vi "GLOBAL_odour_stimuli.vi"() -> ()   [LabVIEW 2016]
panel:
  in  "Odour stimuli":T1(array[cluster])=[{"Name"="UNNAMED2", "Bottles"=[5, 3], "Conc."=1.0, "Unit"=enum."ppm", "Duration"=250.0}, {"Name"="UNNAMED2", "Bottles"=[5, 3], "Conc."=1.0, "Unit"=enum."ppm", "Duration"=250.0}]
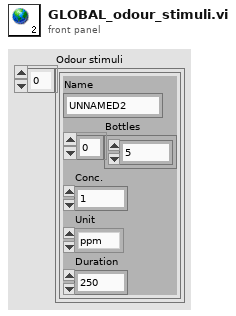
[diagram p1: front panel]
types:
  T1 = cluster{"Name":string, "Bottles":i32[], "Conc.":dbl, "Unit":enum16{"%", "ppm"}, "Duration":dbl}[]
diagram:
